vi "string_binread.vi"(7 "length":i32, 8 "error in":errorcluster caption="エラー入力（エラーなし）", 9 "byte order":T1(ring), 10 "offset":i64, 11 "ref in":refnum<file>) -> (0 "error out":errorcluster caption="エラー出力", 2 "string":string, 3 "ref out":refnum<file>)   [LabVIEW 2015]
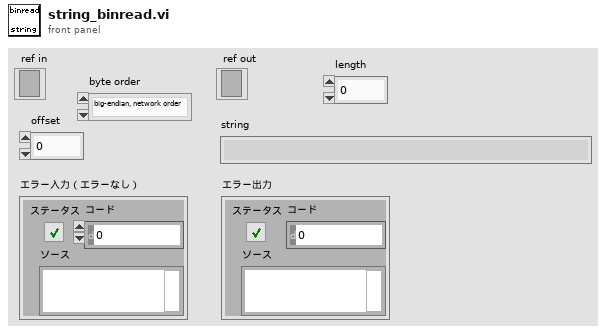
[diagram p1: front panel]
types:
  T1 = enum16{"big-endian, network order", "native, host order", "little-endian"}
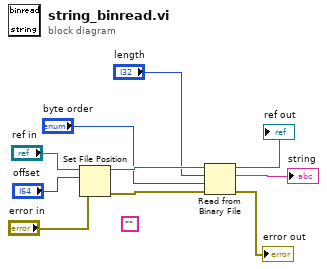
[diagram p0: block diagram]
diagram:
  (unwired) ""
  n1 = Set File Position(offset (in bytes) (0)="offset", refnum="ref in", error in="error in") -> (refnum out=w5:refnum<file>, error out=w6:errorcluster)  [unwired: 1 in]
  n2 = Read from Binary File(8:w6, 9:"byte order", 10:"length", 11:w5) -> (0:→"error out":errorcluster, 2:→"string":string, 3:→"ref out":refnum<file>)  [unwired: 2 in, 1 out]
